vi "DeviceQuery.vi"(4 "error in (no error)":errorcluster, 5 "Command":string, 7 "CmdLib In":refnum<k24>) -> (0 "error out":errorcluster, 1 "Response":string, 3 "CmdLib Out":refnum<k24>)   [LabVIEW 2013]
uses:
  C:/Code/Apps/Utilities/AG-UC2-UC8/AG-UC2-UC8/Install/Samples/LabVIEW/LabVIEW 2013/CmdLibAgilis.dll
  CmdLibAgilis.dll
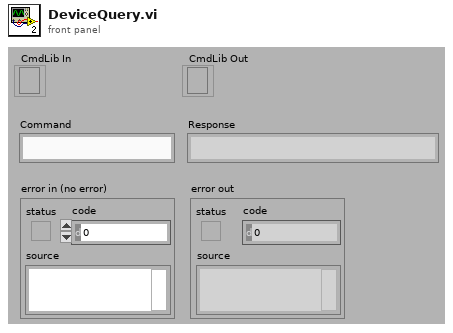
[diagram p1: front panel]
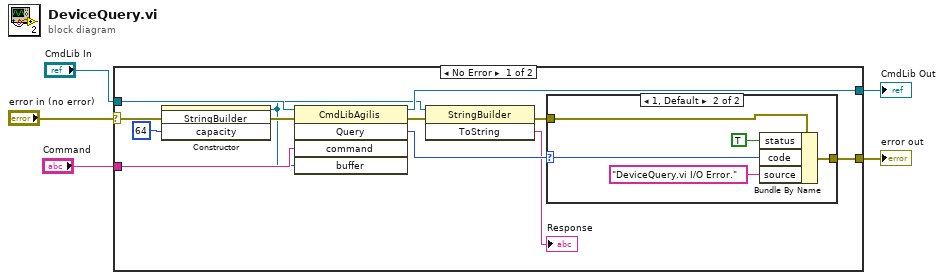
[diagram p0: block diagram]
diagram:
  n1 = case shown="No Error" "error in (no error)" {
    selector: "error in (no error)" -> [w14 w25]
    tunnel: [w9 w25] -> w4
    tunnel: "Command" -> [w7 _]
    tunnel: "CmdLib In" -> [w17 w24]
    tunnel: [w16 w24] -> w1
    frame No Error {
      n2 = constructor class="StringBuilder"(error in=w14, "capacity"=64) -> (reference out=w6:refnum<k24>, error out=w13:errorcluster)  [unwired: 2 in, 2 out]
      n3 = invoke class="CmdLibAgilis" method="Query"(reference=w17, error in=w13, "command"=w7, "buffer"=w6) -> (reference out=w16:refnum<k24>, error out=w12:errorcluster, "Query"=w11:i32)  [unwired: 1 in, 2 out]
      n4 = invoke class="StringBuilder" method="ToString"(reference=w6, error in=w12) -> (error out=w10:errorcluster, "ToString"=→"Response":string)  [unwired: 1 in, 1 out]
      n5 = case shown="1, Default" w11 {
        selector: w11 -> [_ w19]
        tunnel: w10 -> [w18 w21]
        tunnel: [w18 w20] -> w9
        frame 0 {
        }
        frame 1, Default {
          n6 = Bundle By Name(cluster=w21, "status"=TRUE, "code"=w19, "source"="DeviceQuery.vi I/O Error.") -> (w20:errorcluster)
        }
      }
    }
    frame Error {
    }
  }
  "error out" <- w4
  "CmdLib Out" <- w1
